vi "UHR-Fleezers Control (host) - 11.9.vi"() -> ()   [LabVIEW 2014] (continued)
        n1565 = local read "Trap Pos. FB Mult Factor"() -> (w2219:i64)
        n1566 = Add(x=w2222, y=w2220) -> (x+y=w2214:i64)
        n1567 = Multiply(x=32768, y="factor") -> (x*y=w2217:dbl)
        n1568 = Multiply(x=w2217, y=w2219) -> (x*y=w2218:dbl)
        n1569 = Subtract(x=w2214, y=w2218) -> (x-y=w2212:dbl)
        n1570 = To Quad Integer(1:w2212) -> (0:w2213:i64)
        n1571 = xnode "Read/Write Control"("FPGA VI Reference In"=w2226, "error in"=w2225, "Trap Pos. FB Offset Factor"=w2213) -> ()  [unwired: 2 out]
        n1572 = local write "Trap Pos. FB Offset Factor"(w2213) -> ()
      }
      event "Trap Pos. FB Range", "Trap Pos. FB Gains", "Trap Pos. FB Mult Factor", "Trap Pos. FB Offset Factor", "Trap Pos FB Negate Action", "Trap Pos FB Monitor\nT1 or T2", "Differential FB?", "Negate Diff?": Value Change {
        n1573 = event-data() -> ()  [unwired: 7 out]
        n1574 = local read "Negate Diff?"() -> (w2227:bool)
        n1575 = xnode "Read/Write Control"("FPGA VI Reference In"=w2237, "error in"=w2236, "Trap Pos. FB Range"="Trap Pos. FB Range", "Trap Pos. FB Gains"="Trap Pos. FB Gains", "Trap Pos. FB Mult Factor"="Trap Pos. FB Mult Factor", "Trap Pos. FB Offset Factor"="Trap Pos. FB Offset Factor", "Trap Pos FB Negate Action"="Trap Pos FB Negate Action", "Trap Pos FB Monitor T1 or T2"="Trap Pos FB Monitor\nT1 or T2", "AI1 X Scale"="Trap Pos. AI1 X Pre-scale", "Negate Diff?"=w2227, "Diff FB Measurement?"="Differential FB?") -> ()  [unwired: 2 out]
      }
      event "Trap Pos FB SP", "Trap Pos FB SP 2", "Use SP 2": Value Change {
        n1576 = event-data() -> ()  [unwired: 7 out]
        n1577 = Select(t="Trap Pos FB SP 2", s="Use SP 2", f="Trap Pos FB SP") -> (s? t:f=w2238:fxp<+/-,16,1>)
        n1578 = xnode "Read/Write Control"("FPGA VI Reference In"=w2243, "error in"=w2242, "Trap Pos. FB SP"=w2238) -> ()  [unwired: 2 out]
      }
      event "Offset SP2 from SP1": Value Change {
        n1579 = event-data() -> ()  [unwired: 7 out]
        n1580 = local read "Trap Pos FB SP"() -> (w2246:fxp<+/-,16,1>)
        n1581 = Add(x=w2246, y="SP2 Offset") -> (x+y=w2244:fxp<+/-,16,1>)
        n1582 = property on="Trap Pos FB SP 2" class="DigNum (strict)"("Val(Sgnl)"=w2244) -> ()  [unwired: 2 in, 2 out]
        n1583 = local write "Offset SP2 from SP1"(FALSE ("Offset SP2 from SP1")) -> ()
      }
      event "Set Reading to\nSetpoint": Value Change {
        # "This is the actual PID input signal"
        n1584 = event-data() -> ()  [unwired: 7 out]
        n1585 = local write "Set Reading to\nSetpoint"(FALSE ("Set SP to Reading")) -> ()
        n1586 = xnode "Read/Write Control"("FPGA VI Reference In"=w2252, "error in"=w2251) -> ("FPGA VI Reference Out"=w2250:T19, "error out"=w2249:errorcluster, "Trap Pos FB Int-Norm Signal"=w2248:fxp<+/-,16,1>)
        n1587 = local read "Differential FB?"() -> (w2253:bool)
        n1588 = case shown="False" w2253 {
          tunnel: [w2258 w2265] -> w2255
          tunnel: w2248 -> [w2256 w2265]
          frame False {
            n1589 = local read "Trap Pos FB Monitor\nT1 or T2"() -> (w2261:bool)
            n1590 = local read "Trap X AI1 (DMA)"() -> (w2264:T13)
            n1591 = Unbundle By Name(w2264) -> ("Set 1"=w2263:fxp<+/-,16,1>, "Set 2"=w2262:fxp<+/-,16,1>)
            n1592 = Select(t=w2263, s=w2261, f=w2262) -> (s? t:f=w2260:fxp<+/-,16,1>)
            n1593 = Not(x="Set SP Using...") -> (.not. x?=w2257:bool)
            n1594 = Select(t=w2256, s=w2257, f=w2260) -> (s? t:f=w2258:fxp<+/-,16,1>)
          }
          frame True {
          }
        }
        n1595 = xnode "Read/Write Control"("FPGA VI Reference In"=w2250, "error in"=w2249, "Trap Pos. FB SP"=w2255) -> ()  [unwired: 2 out]
        n1596 = local write "Trap Pos FB SP"(w2255) -> ()
      }
      event "Trap Pos. FB Out Scale 2^n": Value Change {
        n1597 = event-data() -> ()  [unwired: 7 out]
        n1598 = Scale By Power Of 2(n="Trap Pos. FB Out Scale 2^n", x=ext 1.0) -> (x*2^n=w2266:ext)
        n1599 = property on="Trap Pos. FB Mult Factor" class="DigNum (strict)"("Val(Sgnl)"=w2266) -> ()  [unwired: 2 in, 2 out]
      }
      event "Trap Pos FB Int Count": Value Change {
        n1600 = event-data() -> ()  [unwired: 7 out]
        n1601 = xnode "Read/Write Control"("FPGA VI Reference In"=w2271, "error in"=w2270, "Trap Pos FB Int Count"="Trap Pos FB Int Count") -> ()  [unwired: 2 out]
      }
      event "Trap pos": Value Change {
        n1602 = event-data() -> ()  [unwired: 7 out]
        n1603 = case shown="True" "Trap pos" {
          frame False {
            n1604 = property on="Trap Delta Graph" class="WFGraph (strict)"("Visible"=TRUE) -> ()  [unwired: 2 in, 2 out]
            n1605 = property on="Saved trap pos" class="WFGraph (strict)"("Visible"=FALSE) -> ()  [unwired: 2 in, 2 out]
          }
          frame True {
            n1606 = property on="Saved trap pos" class="WFGraph (strict)"("Visible"=TRUE) -> ()  [unwired: 2 in, 2 out]
            n1607 = property on="Trap Delta Graph" class="WFGraph (strict)"("Visible"=FALSE) -> ()  [unwired: 2 in, 2 out]
          }
        }
      }
      event "Save user params": Value Change {
        n1608 = event-data() -> ()  [unwired: 7 out]
        n1609 = local write "Save user params"(FALSE ("Save user\nparams")) -> ()
        n1610 = call "save control values.vi"("User"="User") -> ()  [unwired: 8 in, 1 out]
        n1611 = local read "Messages"() -> (w2283:string)
        n1612 = Concatenate Strings("User: ", "User", "\r", "Parameters saved.") -> (w2278:string)
        n1613 = call "Update messages.vi"("Message to add"=w2278, "Old message string"=w2283) -> ("New message string"=w2277:string)
        n1614 = local write "Messages"(w2277) -> ()
      }
      event "Load user params": Value Change {
        n1615 = event-data() -> ()  [unwired: 7 out]
        n1616 = local write "Load user params"(FALSE ("Read user\nparams")) -> ()
        n1617 = flat-sequence {
          tunnel: [w2315] -> w2303
          tunnel: [w2314] -> w2301
          tunnel: [w2313] -> w2299
          tunnel: [w2312] -> w2297
          tunnel: [w2311] -> w2295
          tunnel: [w2310] -> w2293
          tunnel: [w2309] -> w2291
          tunnel: [w2308] -> w2289
          tunnel: [w2307] -> w2287
          tunnel: [w2306] -> w2285
          tunnel: [w2325] -> w2304
          tunnel: w2303 -> [w2325]
          tunnel: [w2324] -> w2302
          tunnel: w2301 -> [w2324]
          tunnel: [w2323] -> w2300
          tunnel: w2299 -> [w2323]
          tunnel: [w2322] -> w2298
          tunnel: w2297 -> [w2322]
          tunnel: [w2321] -> w2296
          tunnel: w2295 -> [w2321]
          tunnel: [w2320] -> w2294
          tunnel: w2293 -> [w2320]
          tunnel: [w2319] -> w2292
          tunnel: w2291 -> [w2319]
          tunnel: [w2318] -> w2290
          tunnel: w2289 -> [w2318]
          tunnel: [w2317] -> w2288
          tunnel: w2287 -> [w2317]
          tunnel: [w2316] -> w2286
          tunnel: w2285 -> [w2316]
          tunnel: w2304 -> [w2342]
          tunnel: w2302 -> [w2341]
          tunnel: w2300 -> [w2340]
          tunnel: w2298 -> [w2339]
          tunnel: w2296 -> [w2338]
          tunnel: w2294 -> [w2337]
          tunnel: w2292 -> [w2336]
          tunnel: w2290 -> [w2335]
          tunnel: w2288 -> [w2334]
          tunnel: w2286 -> [w2333]
          frame #0 {
            # "Make exceptions.\nThese will not be\nloaded."
            n1618 = local read "Sample Channel\nFlow"() -> (w2310:bool)
            n1619 = local read "Green ON/Interlacing"() -> (w2311:bool)
            n1620 = local read "Trap 1 (ON/OFF)"() -> (w2315:bool)
            n1621 = local read "Trap 2 (ON/OFF)"() -> (w2314:bool)
            n1622 = local read "Trap Pos. FB ON"() -> (w2306:bool)
            n1623 = local read "Inject Pump 1"() -> (w2309:bool)
            n1624 = local read "Inject Pump 3"() -> (w2308:bool)
            n1625 = local read "Trap D (MHz)"() -> (w2307:dbl)
            n1626 = local read "Index"() -> (w2312:dbl)
            n1627 = local read "Fish"() -> (w2313:bool)
          }
          frame #1 {
            n1628 = local read "User"() -> (w2326:string)
            n1629 = call "retrieve control values.vi"("User"=w2326) -> ()  [unwired: 10 in, 1 out]
            n1630 = local read "Messages"() -> (w2332:string)
            n1631 = Concatenate Strings("User: ", w2326, "\r", "Parameters loaded.") -> (w2327:string)
            n1632 = call "Update messages.vi"("Message to add"=w2327, "Old message string"=w2332) -> ("New message string"=w2331:string)
            n1633 = local write "Messages"(w2331) -> ()
          }
          frame #2 {
            n1634 = local write "Sample Channel\nFlow"(w2337) -> ()
            n1635 = local write "Green ON/Interlacing"(w2338) -> ()
            n1636 = local write "Trap 1 (ON/OFF)"(w2342) -> ()
            n1637 = local write "Trap 2 (ON/OFF)"(w2341) -> ()
            n1638 = local write "Inject Pump 1"(w2336) -> ()
            n1639 = local write "Trap Pos. FB ON"(w2333) -> ()
            n1640 = local write "Inject Pump 3"(w2335) -> ()
            n1641 = local write "Trap D (MHz)"(w2334) -> ()
            n1642 = local write "Index"(w2339) -> ()
            n1643 = local write "Fish"(w2340) -> ()
          }
        }
      }
      event "Abort wiggle": Value Change {
        n1644 = event-data() -> ()  [unwired: 7 out]
        n1645 = flat-sequence {
          tunnel: w2346 -> [w2350]
          tunnel: w2345 -> [w2349]
          tunnel: [w2348] -> w2343
          tunnel: [w2352] -> w2344
          tunnel: w2343 -> [w2352]
          frame #0 {
            n1646 = xnode "Read/Write Control"("FPGA VI Reference In"=w2350, "error in"=w2349, "Abort wiggle 1"="Abort wiggle", "Abort wiggle 2"="Abort wiggle") -> ("error out"=w2348:errorcluster)  [unwired: 1 out]
          }
          frame #1 {
            n1647 = local write "Abort wiggle"(FALSE ("Abort wiggle")) -> ()
          }
        }
      }
    }
    "error out 2" <- w1148
    n1648 = node-c288() -> ()  [unwired: 2 out]
  }
  n1649 = node-c288() -> (w98:T21)  [unwired: 4 in]
  n1650 = local write "Target size"(cluster{"Width":dbl, "Height":dbl} {"Width"=40.0, "Height"=40.0} ("Target size")) -> ()
  n1651 = timed-loop "Run Scripts, including: stage motion" {
    tunnel: w103 -> [w2360]
    tunnel: w102 -> [w2361]
    tunnel: [w2361] -> w101
    tunnel: [w2360] -> w100
    timing: w98 -> [_]
    timing-out: [_] -> w97
    tunnel: w83 -> [w2359]
    tunnel: w84 -> [w2358]
    tunnel: w24 -> [w2355]
    tunnel: w23 -> [w2354]
    tunnel: w22 -> [w2356]
    tunnel: w21 -> [w2357]
    stop <- w2353 stop-if-true
    n1652 = node-c288() -> ()  [unwired: 1 in, 1 out]
    n1653 = event shown="[3] \"Move Cap. 2 (ADig Top)\": Value Change" {
      selector: _ -> [_ _ _ _ _ _ _ _ _ _ _ _ _ _ _ _ _ _ _ _ _]
      dyn-events: _ -> [_ _ _ _ _ _ _ _ _ _ _ _ _ _ _ _ _ _ _ _ _]
      timeout: _ -> [_ _ _ _ _ _ _ _ _ _ _ _ _ _ _ _ _ _ _ _ _]
      tunnel: ["Set Position" "Move to Position" _ _ "Read Harvard" _ _ _ _ _ _ _ "Got ADig bead" "Force FB Script" "Rupture Script" _ "Got DNA bead" "Take Stepping Data" _ "Take Detection Laser\nImage" _] -> _
      tunnel: [_ _ _ _ _ _ _ _ _ _ _ _ _ _ _ _ _ _ _ _ w3033] -> w2353
      tunnel: w2360 -> [w2379 w2387 w2400 w2430 _ w2478 w2518 w2601 w2632 w2766 w2792 w2827 _ w2844 _ _ _ _ _ _ _]
      tunnel: w2361 -> [w2380 w2388 w2401 w2431 _ w2479 w2519 w2602 w2633 w2767 w2793 w2828 _ w2845 _ _ _ _ _ _ _]
      tunnel: w2359 -> [_ _ _ _ w2463 _ _ _ _ _ _ _ _ _ _ _ _ _ _ _ _]
      tunnel: w2358 -> [_ _ _ _ w2462 _ _ _ _ _ _ _ _ _ _ _ _ _ _ _ _]
      tunnel: w2357 -> [_ _ _ _ _ _ _ _ _ _ _ _ _ _ _ _ _ _ _ _ _]
      tunnel: w2356 -> [_ _ _ _ _ _ _ _ _ _ _ _ _ _ _ _ _ _ _ _ _]
      tunnel: w2355 -> [_ _ _ _ _ _ _ _ _ _ _ _ _ _ _ _ _ _ _ _ _]
      tunnel: w2354 -> [_ _ _ _ _ _ _ _ _ _ _ _ _ _ _ _ _ _ _ _ _]
      event "Set Position", "Set Position 2", "Set Position 3", "Set Position 4", "Set Position 5", "Set Position 1": Value Change {
        n1654 = event-data() -> ()  [unwired: 1 in, 5 out]
        n1655 = Build Array("Set Position 1", "Set Position 2", "Set Position 3", "Set Position 4", "Set Position 5") -> (w2378:bool[])
        n1656 = Boolean Array To Number(Boolean array=w2378) -> (number=w2377:u32)
        n1657 = Logarithm Base 2(1:w2377) -> (0:w2369:dbl)
        n1658 = call "Read Stage Position.vi"("error in"=w2379, "VISA resource name in"=w2380) -> ("Current Position"=w2384:cluster{dbl, dbl, dbl}, "error out"=w2383:errorcluster)  [unwired: 2 out]
        n1659 = Decrement(x="Position") -> (x-1=w2367:dbl)
        n1660 = Greater Or Equal?(x=w2369, y=0.0) -> (x >= y?=w2370:bool)
        n1661 = Cluster To Array(cluster=w2384) -> (array=w2381:dbl[])
        n1662 = local write "Stage Control Serial Error"(w2383) -> ()
        n1663 = Select(t=w2369, s=w2370, f=w2367) -> (s? t:f=w2366:dbl)
        n1664 = Increment(x=w2366) -> (x+1=w2365:dbl)
        n1665 = Build Array (concatenate)(w2365, w2381) -> (w2364:dbl[])
        n1666 = Replace Array Subset(array="Saved Stage Positions", new element=w2364, index (row)=w2366) -> (w2382:dbl[][])  [unwired: 1 in]
        n1667 = local write "Saved Stage Positions"(w2382) -> ()
      }
      event "Move to Position": Value Change {
        n1668 = event-data() -> ()  [unwired: 1 in, 5 out]
        n1669 = flat-sequence {
          tunnel: w2388 -> [w2392]
          tunnel: w2387 -> [w2391]
          frame #0 {
            n1670 = local read "Saved Stage Positions"() -> (w2394:dbl[][])
            n1671 = local read "Position"() -> (w2393:dbl)
            n1672 = local write "Stage Moving"(TRUE ("Stage Moving")) -> ()
            n1673 = call "move to saved stage position.vi"("error in"=w2391, "Stage VISA resource name in"=w2392, "Position"=w2393, "Saved Stage Positions"=w2394) -> ("error out"=w2390:errorcluster)  [unwired: 1 out]
            n1674 = local write "Stage Control Serial Error"(w2390) -> ()
          }
          frame #1 {
            n1675 = call <vilib>:"Beep.vi"() -> ()  [unwired: 3 in, 9 out]
            n1676 = local write "Stage Moving"(FALSE ("Stage Moving")) -> ()
          }
        }
      }
      event "Move Cap. 1 (DNA Bottom)": Value Change {
        n1677 = event-data() -> ()  [unwired: 1 in, 5 out]
        n1678 = local write "Move Cap. 1 (DNA Bottom)"(FALSE ("Move Cap. 1 (DNA Right)")) -> ()
        n1679 = flat-sequence {
          tunnel: w2400 -> [w2403]
          tunnel: w2401 -> [w2404]
          tunnel: [w2404] -> w2398
          tunnel: [w2403] -> w2397
          tunnel: w2398 -> [w2406]
          tunnel: w2397 -> [w2405]
          frame #0 {
            n1680 = property on="Sample Channel\nFlow" class="Bool (strict)"("Val(Sgnl)"="Cap 1 Samp Flow ON") -> ()  [unwired: 2 in, 2 out]
          }
          frame #1 {
            n1681 = local read "Saved Stage Positions"() -> (w2416:dbl[][])
            n1682 = local write "Stage Moving"(TRUE ("Stage Moving")) -> ()
            n1683 = Array Subset(array=w2416, index (row)=0 ("index"), length (row)=1 ("length"), index (col)=1 ("index"), length (col)=3 ("length")) -> (w2413:dbl[][])
            n1684 = Reshape Array(w2413, 3 ("dimension size")) -> (w2411:dbl[])
            n1685 = Array To Cluster(array=w2411) -> (cluster=w2410:cluster{"[0]":dbl, "[1]":dbl, "[2]":dbl})
            n1686 = call "Set Stage Position.vi"("Position"=w2410, "error in"=w2405, "VISA resource name in"=w2406) -> ("error out"=w2409:errorcluster)  [unwired: 2 out]
            n1687 = local write "Stage Control Serial Error"(w2409) -> ()
          }
          frame #2 {
            n1688 = local write "Stage Moving"(FALSE ("Stage Moving")) -> ()
            n1689 = case shown="True" "Cap 1 Flow ON" {
              frame False {
              }
              frame True {
                n1690 = property on="Inject Pump 1" class="Bool (strict)"("Val(Sgnl)"=TRUE ("Value (Signaling)")) -> ()  [unwired: 2 in, 2 out]
              }
            }
            n1691 = call <vilib>:"Beep.vi"() -> ()  [unwired: 3 in, 9 out]
          }
          frame #3 {
            n1692 = property on="Sample Channel\nFlow" class="Bool (strict)"("Val(Sgnl)"=FALSE ("Value (Signaling)")) -> ()  [unwired: 2 in, 2 out]
            n1693 = local read "Cap. 2 BD T1?\n(ADig T1, DNA T2)"() -> (w2423:bool)
            n1694 = case shown="True" w2423 {
              tunnel: "Cap 1 T ON" -> [w2425 w2426]
              frame False {
                n1695 = property on="Trap 1 (ON/OFF)" class="Bool (strict)"("Val(Sgnl)"=w2425) -> ()  [unwired: 2 in, 2 out]
              }
              frame True {
                n1696 = property on="Trap 2 (ON/OFF)" class="Bool (strict)"("Val(Sgnl)"=w2426) -> ()  [unwired: 2 in, 2 out]
              }
            }
            n1697 = property on="Got DNA bead" class="Bool"("Key Focus"=TRUE) -> ()  [unwired: 2 in, 2 out]
          }
        }
      }
      event "Move Cap. 2 (ADig Top)": Value Change {
        n1698 = event-data() -> ()  [unwired: 1 in, 5 out]
        n1699 = local write "Move Cap. 2 (ADig Top)"(FALSE ("Move Cap. 2 (ADig Left)")) -> ()
        n1700 = flat-sequence {
          tunnel: w2430 -> [w2433]
          tunnel: w2431 -> [w2434]
          tunnel: [w2434] -> w2428
          tunnel: [w2433] -> w2427
          tunnel: w2428 -> [w2436]
          tunnel: w2427 -> [w2435]
          frame #0 {
            n1701 = property on="Sample Channel\nFlow" class="Bool (strict)"("Val(Sgnl)"="Cap 2 Samp Flow ON") -> ()  [unwired: 2 in, 2 out]
          }
          frame #1 {
            n1702 = local read "Saved Stage Positions"() -> (w2446:dbl[][])
            n1703 = local write "Stage Moving"(TRUE ("Stage Moving")) -> ()
            n1704 = Array Subset(array=w2446, index (row)=1 ("index"), length (row)=1 ("length"), index (col)=1 ("index"), length (col)=3 ("length")) -> (w2443:dbl[][])
            n1705 = disable-structure shown="Disabled" {
              frame Disabled {
                w2448 = FALSE ("Value (Signaling)")
                n1706 = property on="Trap 1 (ON/OFF)" class="Bool (strict)"("Val(Sgnl)"=w2448) -> ()  [unwired: 2 in, 2 out]
                n1707 = property on="Trap 1 (ON/OFF)" class="Bool (strict)"("Val(Sgnl)"=w2448) -> ()  [unwired: 2 in, 2 out]
              }
              frame Enabled {
              }
            }
            n1708 = Reshape Array(w2443, 3 ("dimension size")) -> (w2441:dbl[])
            n1709 = Array To Cluster(array=w2441) -> (cluster=w2440:cluster{"[0]":dbl, "[1]":dbl, "[2]":dbl})
            n1710 = call "Set Stage Position.vi"("Position"=w2440, "error in"=w2435, "VISA resource name in"=w2436) -> ("error out"=w2439:errorcluster)  [unwired: 2 out]
            n1711 = local write "Stage Control Serial Error"(w2439) -> ()
          }
          frame #2 {
            n1712 = local write "Stage Moving"(FALSE ("Stage Moving")) -> ()
            n1713 = call <vilib>:"Beep.vi"() -> ()  [unwired: 3 in, 9 out]
            n1714 = case shown="True" "Cap 2 Flow ON" {
              frame False {
              }
              frame True {
                n1715 = property on="Inject Pump 3" class="Bool (strict)"("Val(Sgnl)"=TRUE ("Value (Signaling)")) -> ()  [unwired: 2 in, 2 out]
              }
            }
          }
          frame #3 {
            n1716 = Wait (ms)(milliseconds to wait=u32 500) -> ()  [unwired: 1 out]
          }
          frame #4 {
            n1717 = local read "Cal @ (MHz)"() -> (w2454:dbl)
            n1718 = property on="Sample Channel\nFlow" class="Bool (strict)"("Val(Sgnl)"=FALSE ("Value (Signaling)")) -> ()  [unwired: 2 in, 2 out]
            n1719 = case shown="False" "Cap. 2 BD T1?\n(ADig T1, DNA T2)" {
              tunnel: "Cap 2 T ON" -> [w2459 w2460]
              frame False {
                n1720 = property on="Trap 2 (ON/OFF)" class="Bool (strict)"("Val(Sgnl)"=w2459) -> ()  [unwired: 2 in, 2 out]
              }
              frame True {
                n1721 = property on="Trap 1 (ON/OFF)" class="Bool (strict)"("Val(Sgnl)"=w2460) -> ()  [unwired: 2 in, 2 out]
              }
            }
            n1722 = property on="Got ADig bead" class="Bool"("Key Focus"=TRUE) -> ()  [unwired: 2 in, 2 out]
            n1723 = local write "Target"("Target\nON?") -> ()
            n1724 = property on="Trap D (MHz)" class="DigNum (strict)"("Val(Sgnl)"=w2454) -> ()  [unwired: 2 in, 2 out]
          }
        }
      }
      event "Read Harvard": Value Change {
        n1725 = event-data() -> ()  [unwired: 1 in, 5 out]
        n1726 = Concatenate Strings("write buffer", "\r") -> (w2465:string)
        n1727 = VISA Write(VISA resource name=w2463, write buffer=w2465, error in (no error)=w2462) -> (VISA resource name out=w2474:refnum<visa-resource-name>, error out=w2473:errorcluster)  [unwired: 1 out]
        n1728 = stacked-sequence {
          tunnel: [w2477] -> w2472
          tunnel: w2474 -> [w2477]
          tunnel: w2473 -> [w2476]
          tunnel: [w2476] -> w2467
          frame #0 {
            n1729 = Wait (ms)(milliseconds to wait=50) -> ()  [unwired: 1 out]
          }
        }
        n1730 = property class="Instr"(reference=w2472, error in=w2467) -> (reference out=w2471:refnum<visa-resource-name>, error out=w2469:errorcluster, "Serial Settings:Number of Bytes at Serial Port"=w2470:u32)
        "Serial Settings:Number of Bytes at Serial Port" <- w2470
        n1731 = VISA Read(VISA resource name=w2471, byte count=w2470, error in (no error)=w2469) -> (read buffer=w2468:string)  [unwired: 3 out]
        "read buffer" <- w2468
        n1732 = Fract/Exp String To Number(string=w2468) -> ()  [unwired: 5 out]
      }
      event "+z", "-z": Value Change {
        n1733 = event-data() -> ()  [unwired: 1 in, 5 out]
        n1734 = flat-sequence {
          tunnel: w2478 -> [w2500]
          tunnel: w2479 -> [w2480]
          frame #0 {
            n1735 = call "Read Stage Position.vi"("error in"=w2500, "VISA resource name in"=w2480) -> ("Current Position"=w2485:cluster{dbl, dbl, dbl}, "error out"=w2498:errorcluster, "VISA resource name out"=w2499:refnum<visa-resource-name>)  [unwired: 1 out]
            n1736 = local read "Saved Stage Positions"() -> (w2509:dbl[][])
            n1737 = Divide(x="z nudge increment (um)", y=1000.0) -> (x/y=w2497:dbl)
            n1738 = Boolean To (0,1)(Boolean="+z") -> (0, 1=w2489:i16)
            n1739 = Boolean To (0,1)(Boolean="-z") -> (0, 1=w2490:i16)
            n1740 = Array Subset(array=w2509, index (row)=1 ("index"), length (row)=1 ("length"), index (col)=1 ("index"), length (col)=3 ("length")) -> (w2506:dbl[][])
            n1741 = Multiply(x=w2489, y=w2497) -> (x*y=w2493:dbl)
            n1742 = Multiply(x=w2490, y=w2497) -> (x*y=w2491:dbl)
            n1743 = Unbundle(w2485) -> (w2483:dbl, w2482:dbl, w2486:dbl)
            n1744 = Negate(x=w2491) -> (-x=w2492:dbl)
            n1745 = Reshape Array(w2506, 3 ("dimension size")) -> (w2504:dbl[])
            n1746 = Add(x=w2493, y=w2492) -> (x+y=w2494:dbl)
            n1747 = Array To Cluster(array=w2504) -> ()  [unwired: 1 out]
            n1748 = Add(x=w2494, y=w2486) -> (x+y=w2484:dbl)
            n1749 = Bundle(cluster=w2485, w2483, w2482, w2484) -> (w2481:cluster{dbl, dbl, dbl})
            n1750 = call "Set Stage Position.vi"("Position"=w2481, "error in"=w2498, "VISA resource name in"=w2499) -> ("error out"=w2503:errorcluster)  [unwired: 2 out]
            n1751 = local write "Stage Moving"(TRUE ("Stage Moving")) -> ()
            n1752 = local write "Stage Control Serial Error"(w2503) -> ()
          }
          frame #1 {
            n1753 = local write "Stage Moving"(FALSE ("Stage Moving")) -> ()
            n1754 = call <vilib>:"Beep.vi"() -> ()  [unwired: 3 in, 9 out]
          }
        }
      }
      event "Cal/Data Acq. Spot": Value Change {
        n1755 = event-data() -> ()  [unwired: 1 in, 5 out]
        n1756 = flat-sequence {
          tunnel: w2518 -> [w2522]
          tunnel: w2519 -> [w2523]
          tunnel: [w2523] -> w2515
          tunnel: [w2522] -> w2514
          tunnel: w2515 -> [w2528]
          tunnel: w2514 -> [w2527]
          tunnel: ["Cal @ (MHz)"] -> w2512
          tunnel: [w2532] -> w2516
          tunnel: w2512 -> [w2532]
          tunnel: w2516 -> [w2543]
          tunnel: ["W/ Offset 1"] -> w2513
          tunnel: w2516 -> [w2564]
          tunnel: w2513 -> [w2562]
          frame #0 {
            n1757 = property on="Sample Channel\nFlow" class="Bool (strict)"("Val(Sgnl)"="Daq spot flow on") -> ()  [unwired: 2 in, 2 out]
            n1758 = Wait (ms)(milliseconds to wait=u32 250) -> ()  [unwired: 1 out]
          }
          frame #1 {
            n1759 = local read "Saved Stage Positions"() -> (w2525:dbl[][])
            n1760 = property on="Trap D (MHz)" class="DigNum (strict)"("Val(Sgnl)"="Cal @ (MHz)") -> ()  [unwired: 2 in, 2 out]
            n1761 = local write "Stage Moving"(TRUE ("Stage Moving")) -> ()
            n1762 = call "move to saved stage position.vi"("error in"=w2527, "Stage VISA resource name in"=w2528, "Position"="Cal Stage Position", "Saved Stage Positions"=w2525) -> ("error out"=w2526:errorcluster)  [unwired: 1 out]
            n1763 = local write "Stage Control Serial Error"(w2526) -> ()
          }
          frame #2 {
            n1764 = local write "Stage Moving"(FALSE ("Stage Moving")) -> ()
            n1765 = property on="Sample Channel\nFlow" class="Bool (strict)"("Val(Sgnl)"="Flow ON\nduring cal?") -> ()  [unwired: 2 in, 2 out]
            n1766 = call <vilib>:"Beep.vi"() -> ()  [unwired: 3 in, 9 out]
          }
          frame #3 {
            n1767 = local read "Wait Before Save (s)"() -> (w2535:u32)
            n1768 = Multiply(x=w2535, y=u32 1000 ("milliseconds to wait")) -> (x*y=w2536:u32)
            n1769 = Wait (ms)(milliseconds to wait=w2536) -> ()  [unwired: 1 out]
          }
          frame #4 {
            n1770 = property on="Save Calibration" class="Bool (strict)"("Val(Sgnl)"=TRUE ("Value (Signaling)")) -> ()  [unwired: 2 in, 2 out]
          }
          frame #5 {
            n1771 = Wait (ms)(milliseconds to wait=u32 2000) -> ()  [unwired: 1 out]
          }
          frame #6 {
            # "Check to see if \nsaving done"
            n1772 = while {
              stop <- w2539 stop-if-true
              n1773 = local read "Saving..."() -> (w2540:bool)
              n1774 = Wait (ms)(milliseconds to wait=u32 100) -> ()  [unwired: 1 out]
              n1775 = Not(x=w2540) -> (.not. x?=w2539:bool)
            }
          }
          frame #7 {
            n1776 = case shown="True" "W/ Offset 1" {
              tunnel: w2543 -> [_ w2544]
              frame False {
              }
              frame True {
                n1777 = stacked-sequence {
                  tunnel: w2544 -> [_ _ _ _ _ _ _ w2561]
                  frame #0 {
                    n1778 = property on="Trap D (MHz)" class="DigNum (strict)"("Val(Sgnl)"="Offset 1 Start (MHz)") -> ()  [unwired: 2 in, 2 out]
                    n1779 = Replace Array Subset(array=u32[] [0] ("Index Values"), new element="Offset 1 Set", index=0) -> (w2545:u32[])
                    n1780 = property on="Saved AOD Raster Scan Parameter Sets" class="Arr (strict)"("Index Values"=w2545) -> ()  [unwired: 2 in, 2 out]
                  }
                  frame #1 {
                    n1781 = Wait (ms)(milliseconds to wait=u32 200) -> ()  [unwired: 1 out]
                  }
                  frame #2 {
                    n1782 = property on="Load parameters" class="Bool (strict)"("Val(Sgnl)"=TRUE ("Value (Signaling)")) -> ()  [unwired: 2 in, 2 out]
                  }
                  frame #3 {
                    n1783 = Wait (ms)(milliseconds to wait=u32 200) -> ()  [unwired: 1 out]
                  }
                  frame #4 {
                    n1784 = property on="Trap Raster Scan" class="Bool (strict)"("Val(Sgnl)"=TRUE ("Value (Signaling)")) -> ()  [unwired: 2 in, 2 out]
                  }
                  frame #5 {
                    n1785 = Wait (ms)(milliseconds to wait=u32 2000) -> ()  [unwired: 1 out]
                  }
                  frame #6 {
                    n1786 = while {
                      stop <- w2558 stop-if-true
                      n1787 = local read "Raster Scanning..."() -> (w2560:bool)
                      n1788 = local read "Saving..."() -> (w2556:bool)
                      n1789 = Wait (ms)(milliseconds to wait=u32 100) -> ()  [unwired: 1 out]
                      n1790 = Not(x=w2556) -> (.not. x?=w2555:bool)
                      n1791 = Not(x=w2560) -> (.not. x?=w2557:bool)
                      n1792 = And(x=w2557, y=w2555) -> (x .and. y?=w2558:bool)
                    }
                  }
                  frame #7 {
                    n1793 = property on="Trap D (MHz)" class="DigNum (strict)"("Val(Sgnl)"=w2561) -> ()  [unwired: 2 in, 2 out]
                  }
                }
              }
            }
          }
          frame #8 {
            n1794 = local read "Save ave N"() -> (w2563:dbl)
            n1795 = case shown="False" "W/ Offset 2" {
              tunnel: w2564 -> [_ w2571]
              tunnel: w2563 -> [_ w2570]
              tunnel: w2562 -> [w2566 _]
              frame False {
                n1796 = case shown="False" w2566 {
                  frame False {
                    n1797 = Multiply(x="Cal read wait (s)", y=u32 1000 ("milliseconds to wait")) -> (x*y=w2568:u32)
                    n1798 = Wait (ms)(milliseconds to wait=w2568) -> ()  [unwired: 1 out]
                  }
                  frame True {
                  }
                }
              }
              frame True {
                n1799 = stacked-sequence {
                  tunnel: w2571 -> [_ _ _ _ _ _ _ _ _ w2592 _ _]
                  tunnel: w2570 -> [_ _ _ _ _ _ _ _ _ w2590 _ _]
                  frame #0 {
                    n1800 = property on="Save ave N" class="DigNum (strict)"("Val(Sgnl)"=1.0 ("Value (Signaling)")) -> ()  [unwired: 2 in, 2 out]
                  }
                  frame #1 {
                    n1801 = Wait (ms)(milliseconds to wait=u32 500) -> ()  [unwired: 1 out]
                  }
                  frame #2 {
                    n1802 = property on="Trap D (MHz)" class="DigNum (strict)"("Val(Sgnl)"="Offset 2 Start (MHz)") -> ()  [unwired: 2 in, 2 out]
                    n1803 = Replace Array Subset(array=u32[] [0] ("Index Values"), new element="Offset 2 Set", index=0) -> (w2576:u32[])
                    n1804 = property on="Saved AOD Raster Scan Parameter Sets" class="Arr (strict)"("Index Values"=w2576) -> ()  [unwired: 2 in, 2 out]
                  }
                  frame #3 {
                    n1805 = Wait (ms)(milliseconds to wait=u32 500) -> ()  [unwired: 1 out]
                  }
                  frame #4 {
                    n1806 = property on="Load parameters" class="Bool (strict)"("Val(Sgnl)"=TRUE ("Value (Signaling)")) -> ()  [unwired: 2 in, 2 out]
                  }
                  frame #5 {
                    n1807 = Wait (ms)(milliseconds to wait=u32 500) -> ()  [unwired: 1 out]
                  }
                  frame #6 {
                    n1808 = property on="Trap Raster Scan" class="Bool (strict)"("Val(Sgnl)"=TRUE ("Value (Signaling)")) -> ()  [unwired: 2 in, 2 out]
                  }
                  frame #7 {
                    n1809 = Wait (ms)(milliseconds to wait=u32 2000) -> ()  [unwired: 1 out]
                  }
                  frame #8 {
                    n1810 = while {
                      stop <- w2585 stop-if-true
                      n1811 = local read "Raster Scanning..."() -> (w2588:bool)
                      n1812 = local read "Saving..."() -> (w2586:bool)
                      n1813 = Wait (ms)(milliseconds to wait=u32 100) -> ()  [unwired: 1 out]
                      n1814 = Not(x=w2586) -> (.not. x?=w2584:bool)
                      n1815 = Not(x=w2588) -> (.not. x?=w2587:bool)
                      n1816 = And(x=w2587, y=w2584) -> (x .and. y?=w2585:bool)
                    }
                  }
                  frame #9 {
                    n1817 = property on="Trap D (MHz)" class="DigNum (strict)"("Val(Sgnl)"=w2592) -> ()  [unwired: 2 in, 2 out]
                    n1818 = property on="Saved AOD Raster Scan Parameter Sets" class="Arr (strict)"("Index Values"=u32[] [0]) -> ()  [unwired: 2 in, 2 out]
                    n1819 = property on="Save ave N" class="DigNum (strict)"("Val(Sgnl)"=w2590) -> ()  [unwired: 2 in, 2 out]
                  }
                  frame #10 {
                    n1820 = Wait (ms)(milliseconds to wait=u32 500) -> ()  [unwired: 1 out]
                  }
                  frame #11 {
                    n1821 = property on="Load parameters" class="Bool (strict)"("Val(Sgnl)"=TRUE ("Value (Signaling)")) -> ()  [unwired: 2 in, 2 out]
                  }
                }
              }
            }
          }
          frame #9 {
            n1822 = property on="Read Cal" class="Bool (strict)"("Val(Sgnl)"=TRUE ("Value (Signaling)")) -> ()  [unwired: 2 in, 2 out]
          }
          frame #10 {
            n1823 = Wait (ms)(milliseconds to wait=u32 1000) -> ()  [unwired: 1 out]
          }
          frame #11 {
            n1824 = property on="Fish" class="Bool (strict)"("Val(Sgnl)"=TRUE ("Value (Signaling)")) -> ()  [unwired: 2 in, 2 out]
          }
        }
        n1825 = local write "Cal/Data Acq. Spot"(FALSE ("Cal/Data Acq. Spot")) -> ()
      }
      event "Dump Beads": Value Change {
        n1826 = event-data() -> ()  [unwired: 1 in, 5 out]
        n1827 = flat-sequence {
          tunnel: ["Dump spot flow on?"] -> w2598
          tunnel: [w2610] -> w2599
          tunnel: w2598 -> [w2610]
          tunnel: w2602 -> [w2615]
          tunnel: w2601 -> [w2614]
          tunnel: [w2612] -> w2600
          tunnel: w2599 -> [w2612]
          tunnel: w2600 -> [w2626]
          frame #0 {
            w2603 = FALSE ("Value (Signaling)")
            n1828 = local read "Saving..."() -> (w2605:bool)
            n1829 = local write "Dump Beads"(FALSE ("Dump Beads")) -> ()
            n1830 = property on="Inject Pump 3" class="Bool (strict)"("Val(Sgnl)"=w2603) -> ()  [unwired: 2 in, 2 out]
            n1831 = property on="Inject Pump 1" class="Bool (strict)"("Val(Sgnl)"=w2603) -> ()  [unwired: 2 in, 2 out]
            n1832 = local write "Stop Saving"(w2605) -> ()
            n1833 = local write "Fish"(w2603) -> ()
          }
          frame #1 {
            w2606 = TRUE
            w2607 = FALSE ("Fl. Triggered...")
            n1834 = case shown="True" "Dump spot flow on?" {
              frame False {
              }
              frame True {
                n1835 = property on="Sample Channel\nFlow" class="Bool (strict)"("Val(Sgnl)"=TRUE ("Stage Moving")) -> ()  [unwired: 2 in, 2 out]
              }
            }
            n1836 = local write "Fl. Triggered..."(w2607) -> ()
            n1837 = local write "Tether"(w2607) -> ()
            n1838 = local write "Multiple tether"(w2607) -> ()
            n1839 = local write "Good tether"(w2607) -> ()
            n1840 = property on="Green ON/Interlacing" class="Bool (strict)"("Val(Sgnl)"=w2607) -> ()  [unwired: 2 in, 2 out]
            n1841 = property on="Trap Pos. FB ON" class="Bool (strict)"("Val(Sgnl)"=w2607) -> ()  [unwired: 2 in, 2 out]
            n1842 = property on="Trap Trig. Fl." class="Bool (strict)"("Val(Sgnl)"=w2607) -> ()  [unwired: 2 in, 2 out]
            n1843 = local write "Bad fit"(w2607) -> ()
            n1844 = local write "Hysteresis"(w2607) -> ()
            n1845 = property on="Fl. Triggered..." class="Bool (strict)"("Val(Sgnl)"=w2607) -> ()  [unwired: 2 in, 2 out]
            n1846 = local write "Restart DMA? (AOD)"(w2606) -> ()
            n1847 = local write "Save scans"(w2606) -> ()
            n1848 = property on="Dip for Protein" class="Bool (strict)"("Val(Sgnl)"=w2607) -> ()  [unwired: 2 in, 2 out]
            n1849 = property on="Pause dwell" class="Bool (strict)"("Val(Sgnl)"=w2607) -> ()  [unwired: 2 in, 2 out]
          }
          frame #2 {
            n1850 = property on="Trap Pos. FB Offset Factor" class="DigNum (strict)"("Val(Sgnl)"=i64 0 ("Value (Signaling)")) -> ()  [unwired: 2 in, 2 out]
          }
          frame #3 {
            n1851 = local read "Saved Stage Positions"() -> (w2616:dbl[][])
            n1852 = Array Subset(array=w2616, index (row)=3 ("index"), length (row)=1 ("length"), index (col)=1 ("index"), length (col)=3 ("length")) -> (w2621:dbl[][])
            n1853 = local write "Stage Moving"(TRUE ("Stage Moving")) -> ()
            n1854 = Reshape Array(w2621, 3 ("dimension size")) -> (w2619:dbl[])
            n1855 = Array To Cluster(array=w2619) -> (cluster=w2618:cluster{"[0]":dbl, "[1]":dbl, "[2]":dbl})
            n1856 = call "Set Stage Position.vi"("Position"=w2618, "error in"=w2614, "VISA resource name in"=w2615) -> ()  [unwired: 3 out]
          }
          frame #4 {
            w2627 = FALSE ("Value (Signaling)")
            n1857 = case shown="True" w2626 {
              frame False {
              }
              frame True {
                n1858 = property on="Sample Channel\nFlow" class="Bool (strict)"("Val(Sgnl)"=FALSE ("Stage Moving")) -> ()  [unwired: 2 in, 2 out]
              }
            }
            n1859 = property on="Trap 1 (ON/OFF)" class="Bool (strict)"("Val(Sgnl)"=w2627) -> ()  [unwired: 2 in, 2 out]
            n1860 = property on="Trap 2 (ON/OFF)" class="Bool (strict)"("Val(Sgnl)"=w2627) -> ()  [unwired: 2 in, 2 out]
            n1861 = call <vilib>:"Beep.vi"() -> ()  [unwired: 3 in, 9 out]
            n1862 = local write "Fish"(FALSE ("Fish for Tether")) -> ()
          }
          frame #5 {
            n1863 = property on="Move Cap. 2 (ADig Top)" class="Bool (strict)"("Val(Sgnl)"=TRUE ("Value (Signaling)")) -> ()  [unwired: 2 in, 2 out]
            n1864 = property on="Tab Control" class="TabCtl (strict)"("Val(Sgnl)"=T4."Status" ("Value (Signaling)")) -> ()  [unwired: 2 in, 2 out]
          }
        }
      }
      event "Dip for Protein": Value Change {
        n1865 = event-data() -> ()  [unwired: 1 in, 5 out]
        n1866 = case shown="True" "Dip for Protein" {
          tunnel: w2633 -> [_ w2635]
          tunnel: w2632 -> [_ w2634]
          frame False {
          }
          frame True {
            n1867 = while {
              tunnel: w2635 -> [w2646]
              tunnel: w2634 -> [w2645]
              i -> [w2641]
              stop <- w2636 stop-if-true
              n1868 = Increment(x=w2641) -> (x+1=→"Dip #":i32)
              n1869 = flat-sequence {
                tunnel: w2645 -> [w2657]
                tunnel: w2646 -> [w2658]
                tunnel: [w2658] -> w2650
                tunnel: [w2657] -> w2649
                tunnel: [w2651] -> w2637
                tunnel: [w2663] -> w2644
                tunnel: [w2664] -> w2643
                tunnel: w2650 -> [w2665]
                tunnel: w2649 -> [w2666]
                tunnel: [w2661] -> w2638
                tunnel: w2637 -> [w2661]
                tunnel: [w2674] -> w2648
                tunnel: w2644 -> [w2674]
                tunnel: [w2673] -> w2647
                tunnel: w2643 -> [w2673]
                tunnel: [w2670] -> w2642
                tunnel: [w2669] -> w2639
                tunnel: w2638 -> [w2669]
                tunnel: w2647 -> [w2694]
                tunnel: w2648 -> [w2695]
                tunnel: w2642 -> [w2696]
                tunnel: w2639 -> [w2693]
                tunnel: [w2755] -> w2636
                frame #0 {
                  n1870 = local read "Trap Pos. FB ON"() -> (w2651:bool)
                  n1871 = Compound Arithmetic op=AND("Flow ON\nduring dip?", "FB OFF when \nflow ON", w2651) -> (w2652:bool)
                  n1872 = case shown="True" "Move trap \nbefore dip move?" {
                    frame False {
                    }
                    frame True {
                      n1873 = property on="Trap D (MHz)" class="DigNum (strict)"("Val(Sgnl)"="Dipping D (MHz)") -> ()  [unwired: 2 in, 2 out]
                    }
                  }
                  n1874 = property on="Green ON/Interlacing" class="Bool (strict)"("Val(Sgnl)"="Green ON\nbefore dip?") -> ()  [unwired: 2 in, 2 out]
                  n1875 = property on="Sample Channel\nFlow" class="Bool (strict)"("Val(Sgnl)"="Flow ON\nduring dip?") -> ()  [unwired: 2 in, 2 out]
                  n1876 = case shown="True" w2652 {
                    frame False {
                    }
                    frame True {
                      n1877 = property on="Trap Pos. FB ON" class="Bool (strict)"("Val(Sgnl)"=FALSE ("Value (Signaling)")) -> ()  [unwired: 2 in, 2 out]
                    }
                  }
                }
                frame #1 {
                  n1878 = local read "Saved Stage Positions"() -> (w2668:dbl[][])
                  n1879 = local write "Cancel dwell"(FALSE ("Cancel dwell")) -> ()
                  n1880 = call "move to saved stage position.vi"("error in"=w2666, "Stage VISA resource name in"=w2665, "Position"="Dip Stage \nPosition", "Saved Stage Positions"=w2668) -> ("VISA resource name out"=w2663:refnum<visa-resource-name>, "error out"=w2664:errorcluster)
                }
                frame #2 {
                  n1881 = node-c288() -> (w2672:T21)  [unwired: 4 in]
                  n1882 = timed-loop {
                    timing: w2672 -> [_]
                    timing-out: [_] -> w2671
                    tunnel: [w2678] -> w2670
                    i -> [w2675]
                    stop <- w2679 stop-if-true
                    n1883 = node-c288() -> ()  [unwired: 1 in, 1 out]
                    n1884 = Greater Or Equal?(x=w2675, y="Dip Duration (s)") -> (x >= y?=w2687:bool)
                    n1885 = local read "Dip for Protein"() -> (w2680:bool)
                    n1886 = local read "Dump Beads"() -> (w2677:bool)
                    n1887 = local read "Cancel dwell"() -> (w2686:bool)
                    n1888 = local read "Pause dwell"() -> (w2683:bool)
                    n1889 = Not(x=w2680) -> (.not. x?=w2685:bool)
                    n1890 = Compound Arithmetic op=OR(w2686, w2687, w2685) -> (w2684:bool)
                    n1891 = Select(t=FALSE, s=w2683, f=w2684) -> (s? t:f=w2681:bool)
                    n1892 = Not(x=w2677) -> (.not. x?=w2676:bool)
                    n1893 = node-c288() -> ()  [unwired: 1 in, 1 out]
                    n1894 = And(x=w2680, y=w2676) -> (x .and. y?=w2678:bool)
                    n1895 = Or(x=w2681, y=w2677) -> (x .or. y?=w2679:bool)
                    "Dip Time (s)" <- w2675
                  }
                  n1896 = node-c288(w2671) -> ()  [unwired: 1 out]
                }
                frame #3 {
                  n1897 = case shown="True" w2696 {
                    tunnel: w2695 -> [_ w2701]
                    tunnel: w2694 -> [_ w2700]
                    tunnel: w2693 -> [_ w2697]
                    frame False {
                    }
                    frame True {
                      n1898 = flat-sequence {
                        tunnel: w2700 -> [w2705]
                        tunnel: w2701 -> [w2706]
                        tunnel: [w2706] -> w2699
                        tunnel: [w2705] -> w2698
                        tunnel: w2697 -> [w2702]
                        tunnel: w2699 -> [w2716]
                        tunnel: w2698 -> [w2715]
                        tunnel: w2697 -> [w2724]
                        frame #0 {
                          n1899 = local read "Sample Channel\nFlow"() -> (w2704:bool)
                          n1900 = case shown="True" w2704 {
                            tunnel: "Flow ON \nduring return\nfrom dip?" -> [w2707 w2710]
                            tunnel: w2702 -> [_ w2709]
                            frame False {
                              n1901 = case shown="True" w2707 {
                                frame False {
                                }
                                frame True {
                                n1902 = property on="Sample Channel\nFlow" class="Bool (strict)"("Val(Sgnl)"=TRUE ("Value (Signaling)")) -> ()  [unwired: 2 in, 2 out]
                                }
                              }
                            }
                            frame True {
                              n1903 = case shown="False" w2710 {
                                tunnel: w2709 -> [w2711 _]
                                frame False {
                                n1904 = property on="Trap Pos. FB ON" class="Bool (strict)"("Val(Sgnl)"=w2711) -> ()  [unwired: 2 in, 2 out]
                                n1905 = property on="Sample Channel\nFlow" class="Bool (strict)"("Val(Sgnl)"=FALSE ("Value (Signaling)")) -> ()  [unwired: 2 in, 2 out]
                                }
                                frame True {
                                }
                              }
                            }
                          }
                        }
                        frame #1 {
                          # "For turning on green laser before stage reaches lower spot"
                          n1906 = case shown="True" "Green ON\nafter start\nreturn?" {
                            frame False {
                            }
                            frame True {
                              n1907 = flat-sequence {
                                frame #0 {
                                n1908 = Multiply(x="Green delay after \nstart return (s)", y=1000.0) -> (x*y=w2721:dbl)
                                n1909 = Wait (ms)(milliseconds to wait=w2721) -> ()  [unwired: 1 out]
                                }
                                frame #1 {
                                n1910 = property on="Green ON/Interlacing" class="Bool (strict)"("Val(Sgnl)"=TRUE ("Value (Signaling)")) -> ()  [unwired: 2 in, 2 out]
                                }
                              }
                            }
                          }
                          n1911 = local read "Saved Stage Positions"() -> (w2719:dbl[][])
                          n1912 = local write "Cancel dwell"(FALSE ("Cancel dwell")) -> ()
                          n1913 = call "move to saved stage position.vi"("error in"=w2715, "Stage VISA resource name in"=w2716, "Position"="Return Stage \nPosition", "Saved Stage Positions"=w2719) -> ("error out"=w2717:errorcluster)  [unwired: 1 out]
                          n1914 = local write "Stage Control Serial Error"(w2717) -> ()
                        }
                        frame #2 {
                          n1915 = property on="Trap Pos. FB ON" class="Bool (strict)"("Val(Sgnl)"=w2724) -> ()  [unwired: 2 in, 2 out]
                          n1916 = case shown="True" "Green ON \nafter return?" {
                            frame False {
                            }
                            frame True {
                              n1917 = property on="Green ON/Interlacing" class="Bool (strict)"("Val(Sgnl)"=TRUE ("Value (Signaling)")) -> ()  [unwired: 2 in, 2 out]
                            }
                          }
                          n1918 = case shown="True" "Move trap after return?" {
                            frame False {
                            }
                            frame True {
                              n1919 = property on="Trap D (MHz)" class="DigNum (strict)"("Val(Sgnl)"="Dip Trap D 2 (MHz)") -> ()  [unwired: 2 in, 2 out]
                            }
                          }
                          n1920 = case shown="True" "Save data after return?" {
                            frame False {
                            }
                            frame True {
                              n1921 = property on="Start Saving" class="Bool (strict)"("Val(Sgnl)"=TRUE ("Value (Signaling)")) -> ()  [unwired: 2 in, 2 out]
                            }
                          }
                          n1922 = property on="Sample Channel\nFlow" class="Bool (strict)"("Val(Sgnl)"="Flow ON\nduring daq?") -> ()  [unwired: 2 in, 2 out]
                        }
                        frame #3 {
                          n1923 = node-c288() -> (w2733:T21)  [unwired: 4 in]
                          n1924 = timed-loop {
                            timing: w2733 -> [_]
                            timing-out: [_] -> w2732
                            i -> [w2734]
                            stop <- w2736 stop-if-true
                            n1925 = node-c288() -> ()  [unwired: 1 in, 1 out]
                            n1926 = local read "Dump Beads"() -> (w2735:bool)
                            n1927 = Greater Or Equal?(x=w2734, y="Dwell Duration (s)") -> (x >= y?=w2741:bool)
                            n1928 = local read "Dip for Protein"() -> (w2738:bool)
                            n1929 = Not(x=w2738) -> (.not. x?=w2737:bool)
                            n1930 = Compound Arithmetic op=OR(w2741, "Cancel dwell", w2737) -> (w2740:bool)
                            n1931 = node-c288() -> ()  [unwired: 1 in, 1 out]
                            n1932 = Select(t=FALSE, s="Pause dwell", f=w2740) -> (s? t:f=w2743:bool)
                            n1933 = Or(x=w2743, y=w2735) -> (x .or. y?=w2736:bool)
                            "Dwell Time (s)" <- w2734
                          }
                          n1934 = node-c288(w2732) -> ()  [unwired: 1 out]
                        }
                      }
                    }
                  }
                }
                frame #4 {
                  n1935 = local read "Dip for Protein"() -> (w2752:bool)
                  n1936 = local read "Tether"() -> (w2751:bool)
                  n1937 = local read "Dump Beads"() -> (w2753:bool)
                  n1938 = local write "Cancel dwell"(FALSE ("Cancel dwell")) -> ()
                  n1939 = Not(x=w2751) -> (.not. x?=w2750:bool)
                  n1940 = Not(x=w2752) -> (.not. x?=w2756:bool)
                  n1941 = Not(x="Cont. Repeat Dipping?") -> (.not. x?=w2758:bool)
                  n1942 = Compound Arithmetic op=OR(w2750, w2756, w2758, w2753) -> (w2755:bool)
                }
              }
            }
          }
        }
      }
      event "Profile": Value Change {
        n1943 = event-data() -> ()  [unwired: 1 in, 5 out]
        n1944 = flat-sequence {
          tunnel: w2767 -> [w2770]
          tunnel: w2766 -> [w2778]
          tunnel: [w2772] -> w2765
          tunnel: [w2771] -> w2764
          tunnel: [w2769] -> w2762
          tunnel: [w2768] -> w2759
          tunnel: w2765 -> [w2785]
          tunnel: w2764 -> [w2784]
          tunnel: [w2782] -> w2763
          tunnel: w2762 -> [w2783]
          tunnel: [w2781] -> w2761
          tunnel: [w2780] -> w2760
          tunnel: w2759 -> [w2780]
          tunnel: w2763 -> [w2789]
          tunnel: w2761 -> [w2788]
          tunnel: w2760 -> [w2787]
          frame #0 {
            n1945 = call "Read Stage Position.vi"("error in"=w2778, "VISA resource name in"=w2770) -> ("Current Position"=w2768:cluster{dbl, dbl, dbl}, "error out"=w2771:errorcluster, "VISA resource name out"=w2769:refnum<visa-resource-name>)  [unwired: 1 out]
            "Current Position" <- w2768
            n1946 = local write "Stage Control Serial Error"(w2771) -> ()
            n1947 = Unbundle(w2768) -> (w2775:dbl, w2777:dbl, w2773:dbl)
            n1948 = Add(x=w2777, y="Y change (mm)") -> (x+y=w2774:dbl)
            n1949 = Bundle(w2775, w2774, w2773) -> (w2772:cluster{dbl, dbl, dbl})  [unwired: 1 in]
          }
          frame #1 {
            # "move to new position and start saving"
            n1950 = local write "Stage Moving"(TRUE ("Stage Moving")) -> ()
            n1951 = local write "Start Saving"(TRUE ("Start Saving")) -> ()
            n1952 = call "Set Stage Position.vi"("Position"=w2785, "error in"=w2784, "VISA resource name in"=w2783) -> ("error out"=w2781:errorcluster, "VISA resource name out"=w2782:refnum<visa-resource-name>)  [unwired: 1 out]
          }
          frame #2 {
            # "go back to start"
            n1953 = call "Set Stage Position.vi"("Position"=w2787, "error in"=w2788, "VISA resource name in"=w2789) -> ()  [unwired: 3 out]
          }
          frame #3 {
            # "stop saving"
            n1954 = local write "Stop Saving"(TRUE ("Stop Saving")) -> ()
            n1955 = local write "Stage Moving"(FALSE ("Stage Moving")) -> ()
          }
        }
      }
      event "Move to Position 1", "Move to Position 2", "Move to Position 3", "Move to Position 4", "Move to Position 5", "Lower Ch. Cap.": Value Change {
        n1956 = event-data() -> ()  [unwired: 1 in, 5 out]
        n1957 = Or(x="Move to Position 5", y="Lower Ch. Cap.") -> (x .or. y?=w2795:bool)
        n1958 = Build Array("Move to Position 1", "Move to Position 2", "Move to Position 3", "Move to Position 4", w2795) -> (w2798:bool[])
        n1959 = Boolean Array To Number(Boolean array=w2798) -> (number=w2797:u32)
        n1960 = Logarithm Base 2(1:w2797) -> (0:w2796:dbl)
        n1961 = flat-sequence {
          tunnel: w2796 -> [w2807]
          tunnel: w2793 -> [w2805]
          tunnel: w2792 -> [w2804]
          frame #0 {
            n1962 = local read "Saved Stage Positions"() -> (w2815:dbl[][])
            n1963 = Array Subset(array=w2815, index (row)=w2807, length (row)=1 ("length"), index (col)=1 ("index"), length (col)=3 ("length")) -> (w2812:dbl[][])
